vi "CSM Part Property at Cursor.vi"(9 "Pos":i32, 11 "Single-line Text":string) -> (0 "Msg Type":T3, 1 "Array":i32[](array[numeric]), 3 "Property":T1[](array[typedef]))   [LabVIEW 2017]
uses:
  Single-Line Type.ctl
  CSM Part Property.ctl
  Single-Line Selection Type.ctl
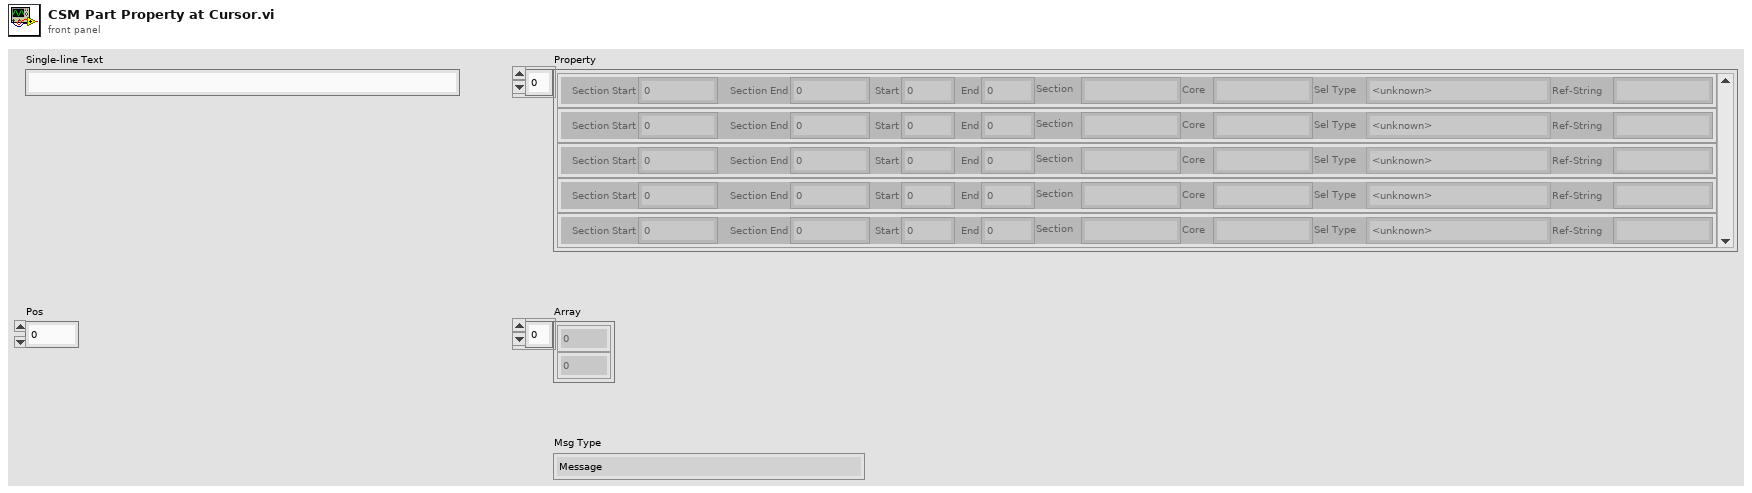
[diagram p1: front panel]
types:
  T1 = typedef "CSM Part Property.ctl" = cluster{"Section Start":u32, "Section End":u32, "Start":u32, "End":u32, "Section":string, "Core":string, "Sel Type":T2, "Ref-String":string}
  T2 = typedef "Single-Line Selection Type.ctl" = enum16{"<unknown>", "Reg-SourceSignal", "Reg-@Seperator", "Reg-ArgSymbol", "Reg-TargetAPI", "Reg-Module", "Reg-Symbol", "Reg-Oper", "Msg-State", "Msg-Arg", "Msg-ArgSymbol", "Msg-Symbol", "Msg-Module", "Broadcast-Signal", "Broadcast-ArgSymbol", "Broadcast-Arg", "Broadcast-Symbol", "Broadcast-Oper", "Comment-Symbol", "Comment-Content"}
  T3 = typedef "Single-Line Type.ctl" = enum16{"Message", "Broadcast", "Registration"}
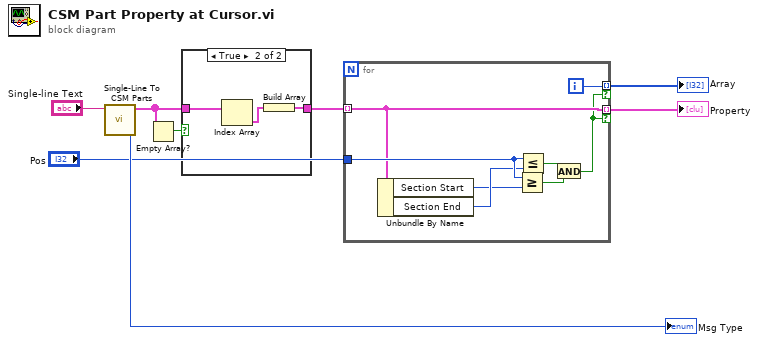
[diagram p0: block diagram]
diagram:
  n1 = call "Single-Line To CSM Parts.vi"("Single-line Text"="Single-line Text") -> ("Msg Type"=→"Msg Type":T3, "Property"=w1:T1[])  [unwired: 7 in, 2 out]
  n2 = Empty Array?(array=w1) -> (empty?=w3:bool)
  n3 = case shown="True" w3 {
    tunnel: [w9 w11] -> w2
    tunnel: w1 -> [w9 w12]
    frame False {
    }
    frame True {
      n4 = Index Array(array=w12) -> (element=w10:T1)  [unwired: 1 in]
      n5 = Build Array(w10) -> (w11:T1[])
    }
  }
  n6 = for {
    tunnel: "Pos" -> [w20]
    tunnel: w2 -> [w15] mode=indexing
    tunnel: [w15] -> w4 mode=indexing if=w13
    tunnel: [w14] -> w5 mode=indexing if=w13
    i -> [w14]
    n7 = Unbundle By Name(w15) -> ("Section Start"=w16:u32, "Section End"=w17:u32)
    n8 = Greater Or Equal?(x=w20, y=w16) -> (x >= y?=w18:bool)
    n9 = Less Or Equal?(x=w20, y=w17) -> (x <= y?=w19:bool)
    n10 = And(x=w19, y=w18) -> (x .and. y?=w13:bool)
  }
  "Property" <- w4
  "Array" <- w5
